vi "Configuration - Load Carrier Settings.vi"(7 "Section":string, 8 "error in":errorcluster, 11 "Refnum in":T1) -> (0 "error out":errorcluster, 3 "refnum out":T1)   [LabVIEW 2017, in "Communications Library.lvlib"]
uses:
  Communications Library.lvlib
  <vilib>/Utility/config.llb/Config Data RefNum.ctl
  Typedefs/DTACQ Module Carrier Configuration--Cluster.ctl
  Typedefs/DTACQ Module Configuration--Cluster.ctl
  Typedefs/DTACQ Device Type--Enum.ctl
  Typedefs/Functional Global Variable Action--Enum.ctl
  <vilib>/Utility/config.llb/Read Key (String).vi
  <vilib>/Utility/config.llb/Read Key (I32).vi
  <vilib>/Utility/config.llb/NI_LVConfig.lvlib
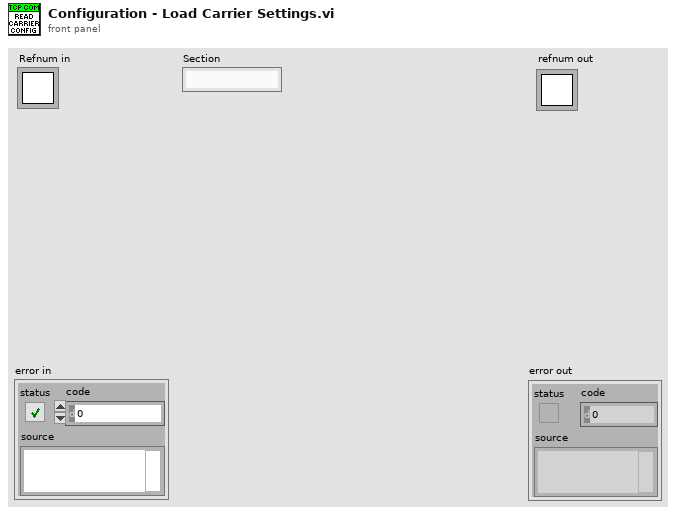
[diagram p1: front panel]
types:
  T1 = typedef "NI_LVConfig.lvlib/Config Data RefNum.ctl" = refnum<k1>
  T2 = typedef "Communications Library.lvlib/Functional Global Variable Action--Enum.ctl" = enum16{"Initialise", "Write Module Config", "Write Carrier Config", "Read"}
  T3 = typedef "Communications Library.lvlib/DTACQ Module Carrier Configuration--Cluster.ctl" = cluster{"Name":string, "IP":string, "Control Port":i32, "Timeout (ms)":i32, "Continuous Capture Port (Multiplexed)":i32, "Start HIL Shot Port":i32, "AWG Upload Port (Multiplexed)":i32, "Download Captured Data Port (Multiplexed)":i32, "Module Slots":i32, "Module Configurations":T4[]}
  T4 = typedef "Communications Library.lvlib/DTACQ Module Configuration--Cluster.ctl" = cluster{"Name":string, "Position":string, "Module Type":T5, "Control Port":i32, "Timeout (ms)":i32, "Channels":i32}
  T5 = typedef "Communications Library.lvlib/DTACQ Device Type--Enum.ctl" = enum16{"Carrier", "Analog In Module", "Analog Out Module", "Generic Module"}
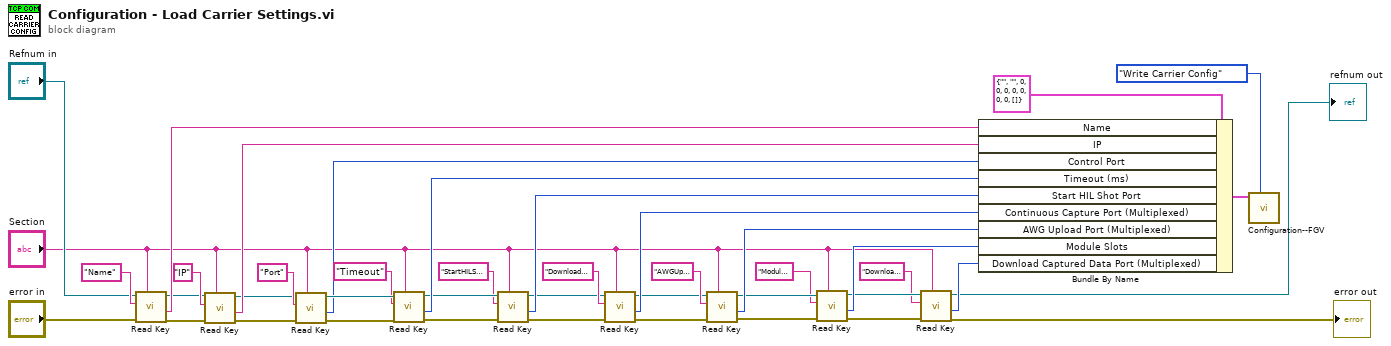
[diagram p0: block diagram]
diagram:
  n1 = call-poly <vilib>:"Read Key.vi"("section"="Section", "error in (no error)"="error in", "key"="Name", "refnum"="Refnum in") -> ("error out"=w16:errorcluster, "value"=w30:string, "refnum out"=w17:T1)  [unwired: 4 in, 1 out]
  n2 = call-poly <vilib>:"Read Key.vi"("section"="Section", "error in (no error)"=w16, "key"="IP", "refnum"=w17) -> ("error out"=w18:errorcluster, "value"=w31:string, "refnum out"=w19:T1)  [unwired: 4 in, 1 out]
  n3 = call-poly <vilib>:"Read Key.vi"("section"="Section", "error in (no error)"=w18, "key"="Port", "refnum"=w19) -> ("error out"=w37:errorcluster, "value"=w32:i32, "refnum out"=w38:T1)  [unwired: 4 in, 1 out]
  n4 = call-poly <vilib>:"Read Key.vi"("section"="Section", "error in (no error)"=w37, "key"="Timeout", "refnum"=w38) -> ("error out"=w40:errorcluster, "value"=w41:i32, "refnum out"=w39:T1)  [unwired: 4 in, 1 out]
  n5 = call-poly <vilib>:"Read Key.vi"("section"="Section", "error in (no error)"=w40, "key"="StartHILShotPort", "refnum"=w39) -> ("error out"=w26:errorcluster, "value"=w34:i32, "refnum out"=w23:T1)  [unwired: 4 in, 1 out]
  n6 = call-poly <vilib>:"Read Key.vi"("section"="Section", "error in (no error)"=w26, "key"="DownloadContinuousDataPortMux", "refnum"=w23) -> ("error out"=w25:errorcluster, "value"=w35:i32, "refnum out"=w24:T1)  [unwired: 4 in, 1 out]
  n7 = call-poly <vilib>:"Read Key.vi"("section"="Section", "error in (no error)"=w25, "key"="AWGUploadPortMux", "refnum"=w24) -> ("error out"=w10:errorcluster, "value"=w33:i32, "refnum out"=w11:T1)  [unwired: 4 in, 1 out]
  n8 = call-poly <vilib>:"Read Key.vi"("section"="Section", "error in (no error)"=w10, "key"="ModuleSlots" ("section"), "refnum"=w11) -> ("error out"=w7:errorcluster, "value"=w9:i32, "refnum out"=w6:T1)  [unwired: 4 in, 1 out]
  n9 = call-poly <vilib>:"Read Key.vi"("section"="Section", "error in (no error)"=w7, "key"="DownloadCapturedDataPortMux", "refnum"=w6) -> ("error out"=→"error out":errorcluster, "value"=w5:i32, "refnum out"=→"refnum out":T1)  [unwired: 4 in, 1 out]
  n10 = Bundle By Name(cluster=T3 {"Name"="", "IP"="", "Control Port"=0, "Timeout (ms)"=0, "Continuous Capture Port (Multiplexed)"=0, "Start HIL Shot Port"=0, "AWG Upload Port (Multiplexed)"=0, "Download Captured Data Port (Multiplexed)"=0, "Module Slots"=0, "Module Configurations"=[]} ("DTACQ Module Carrier Configuration"), "Name"=w30, "IP"=w31, "Control Port"=w32, "Timeout (ms)"=w41, "Start HIL Shot Port"=w34, "Continuous Capture Port (Multiplexed)"=w35, "AWG Upload Port (Multiplexed)"=w33, "Module Slots"=w9, "Download Captured Data Port (Multiplexed)"=w5) -> (w13:T3)
  n11 = call "Configuration--FGV.vi"("Functional Global Action"=Functional_Global_Variable_Action--Enum."Write Carrier Config", "Carrier Configuration In"=w13) -> ()  [unwired: 8 in, 2 out]
